vi "Build_Asylum_SetOutWave.vi"(6 "interpolation":i32, 8 "error in (no error)":errorcluster, 9 "Wave":cluster{"channelString":string, "wave":string}, 10 "eventString":string, 11 "whichBank":i32) -> (0 "error out":errorcluster, 3 "Command":string)   [LabVIEW 2020]
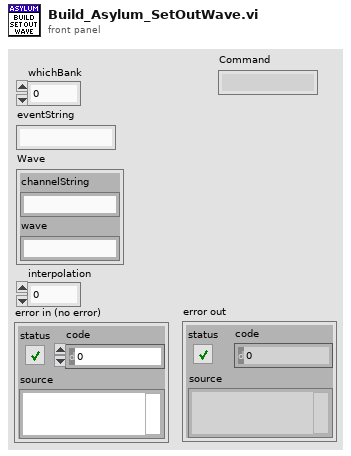
[diagram p1: front panel]
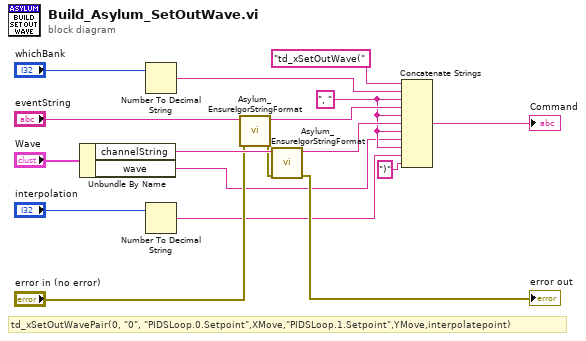
[diagram p0: block diagram]
diagram:
  w5 = ", " ("string")
  # "td_xSetOutWavePair(0, \"0\", \"PIDSLoop.0.Setpoint\",XMove,\"PIDSLoop.1.Setpoint\",YMove,interpolatepoint)"
  n1 = Unbundle By Name("Wave") -> ("channelString"=w13:string, "wave"=w1:string)
  n2 = Number To Decimal String(number="whichBank") -> (decimal integer string=w8:string)  [unwired: 1 in]
  n3 = Number To Decimal String(number="interpolation") -> (decimal integer string=w4:string)  [unwired: 1 in]
  n4 = call "Asylum_EnsureIgorStringFormat.vi"("error in (no error)"="error in (no error)", "Value"="eventString") -> ("error out"=w12:errorcluster, "Value"=w7:string)  [unwired: 8 in]
  n5 = call "Asylum_EnsureIgorStringFormat.vi"("error in (no error)"=w12, "Value"=w13) -> ("error out"=→"error out":errorcluster, "Value"=w6:string)  [unwired: 8 in]
  n6 = Concatenate Strings("td_xSetOutWave(" ("string"), w8, w5, w7, w5, w6, w5, w1, w5, w4, ")" ("string")) -> (→"Command":string)
